vi "Monitoring task.vi"   [LabVIEW 2022 SP3]
uses:
  PLC/PLC.lvlib
types:
  T1 = cluster{bool, "测试模式":enum16{"水样测试", "平行样测试", "集成干预测试", "加标回收"}}
  T2 = typedef "启动参数.ctl" = cluster{"氨氮":bool, "总磷":bool, "总氮":bool, "多参数":bool, "CODmn":bool, "CODCr":bool, "氟化物":bool, "超标留样":bool, "重金属":bool, "挥发酚":bool, "综合生物毒性":bool}
  T3 = cluster{"控制命令":enum16{"启动测量", "标样核查", "零点核查", "跨度核查", "空白测试", "平行样测试", "加标回收", "空白校准", "标样校准", "初始化（清洗）", "停止测试", "仪器重启", "校时", "模式设置", "测量间隔设置"}, "自动运行启动参数":T2}
  T4 = typedef "参数.ctl" = cluster{"测试模式":enum16{"水样测试", "平行样测试", "集成干预测试", "加标回收"}, "参数启用":T2}
  T5 = enum16{"空闲", "润洗", "采样", "沉淀", "配水", "反冲洗", "储水", "结束"}
  T6 = typedef "控制命令与参数.ctl" = cluster{"控制命令":enum16{"启动测量", "标样核查", "零点核查", "跨度核查", "空白测试", "平行样测试", "加标回收", "空白校准", "标样校准", "初始化（清洗）", "停止测试", "仪器重启", "校时", "模式设置", "测量间隔设置"}, "测量参数":string}
  T7 = enum16{"启动测量", "标样核查", "零点核查", "跨度核查", "空白测试", "平行样测试", "加标回收", "空白校准", "标样校准", "初始化（清洗）", "停止测试", "仪器重启", "校时", "模式设置", "测量间隔设置"}
  T8 = typedef "斯坦道原位多参数.lvlib/水样测试启动自定义输入参数.ctl" = cluster{"测量模式":string, "数据类型":string}
  T9 = typedef "多参数模块版本.ctl" = enum16{"原位多参数", "集成式多参"}
  T10 = cluster{"系统时间":timestamp, "工作状态":u16, "测量模式":u16, "告警代码":enum16{"无告警", "缺试剂告警", "缺水样告警", "缺蒸馏水告警", "缺标液告警", "仪表漏液告警", "标定异常告警", "超量程告警", "加热异常", "低试剂预警", "超上限告警", "超下限告警", "仪表内部其他异常", "滴定异常告警", "电极异常告警", "量程切换告警", "参数设置告警", "PH电极电位异常", "电导率电极异常", "浊度光度异常", "溶解氧电极异常", "溶解氧光强异常", "温度异常告警", "PH异常告警", "溶解氧异常告警", "电导率异常告警", "浊度异常告警", "叶绿素异常告警", "藻密度异常告警", "蓝绿藻异常告警", "ORP异常告警", "氨氮异常告警", "清洁刷异常告警", "SD卡异常告警", "蓝牙异常告警", "Wifi异常告警", "流程异常告警"}, "故障代码":enum16{"无故障", "电机故障", "温度故障", "通讯故障", "滴定故障"}, "日志代码":u16, "软件版本":string}
  T11 = cluster{"命令":string, "测量模式":enum16{"水样测量", "标样核查", "零点核查", "跨度核查", "空白测试", "加标回收", "平行样", "校零", "校标"}, "CODMn量程切换":enum32{"H", "L", "AUTO"}}
  T12 = enum16{"水样测量", "标样核查", "零点核查", "跨度核查", "空白测试", "加标回收", "平行样", "校零", "校标"}
  T13 = typedef "模块配置类型.ctl" = enum16{"单模块", "总磷总氮二合一模块", "氨氮总磷二合一模块"}
  T14 = typedef "CODMn模块版本.ctl" = enum16{"PLC版", "单片机版", "通用流路版本"}
  T15 = typedef "CODcr模块版本.ctl" = enum16{"斯坦道V3", "点创"}
  T16 = typedef "氨氮总磷总氮模块版本.ctl" = enum16{"V2", "V3"}
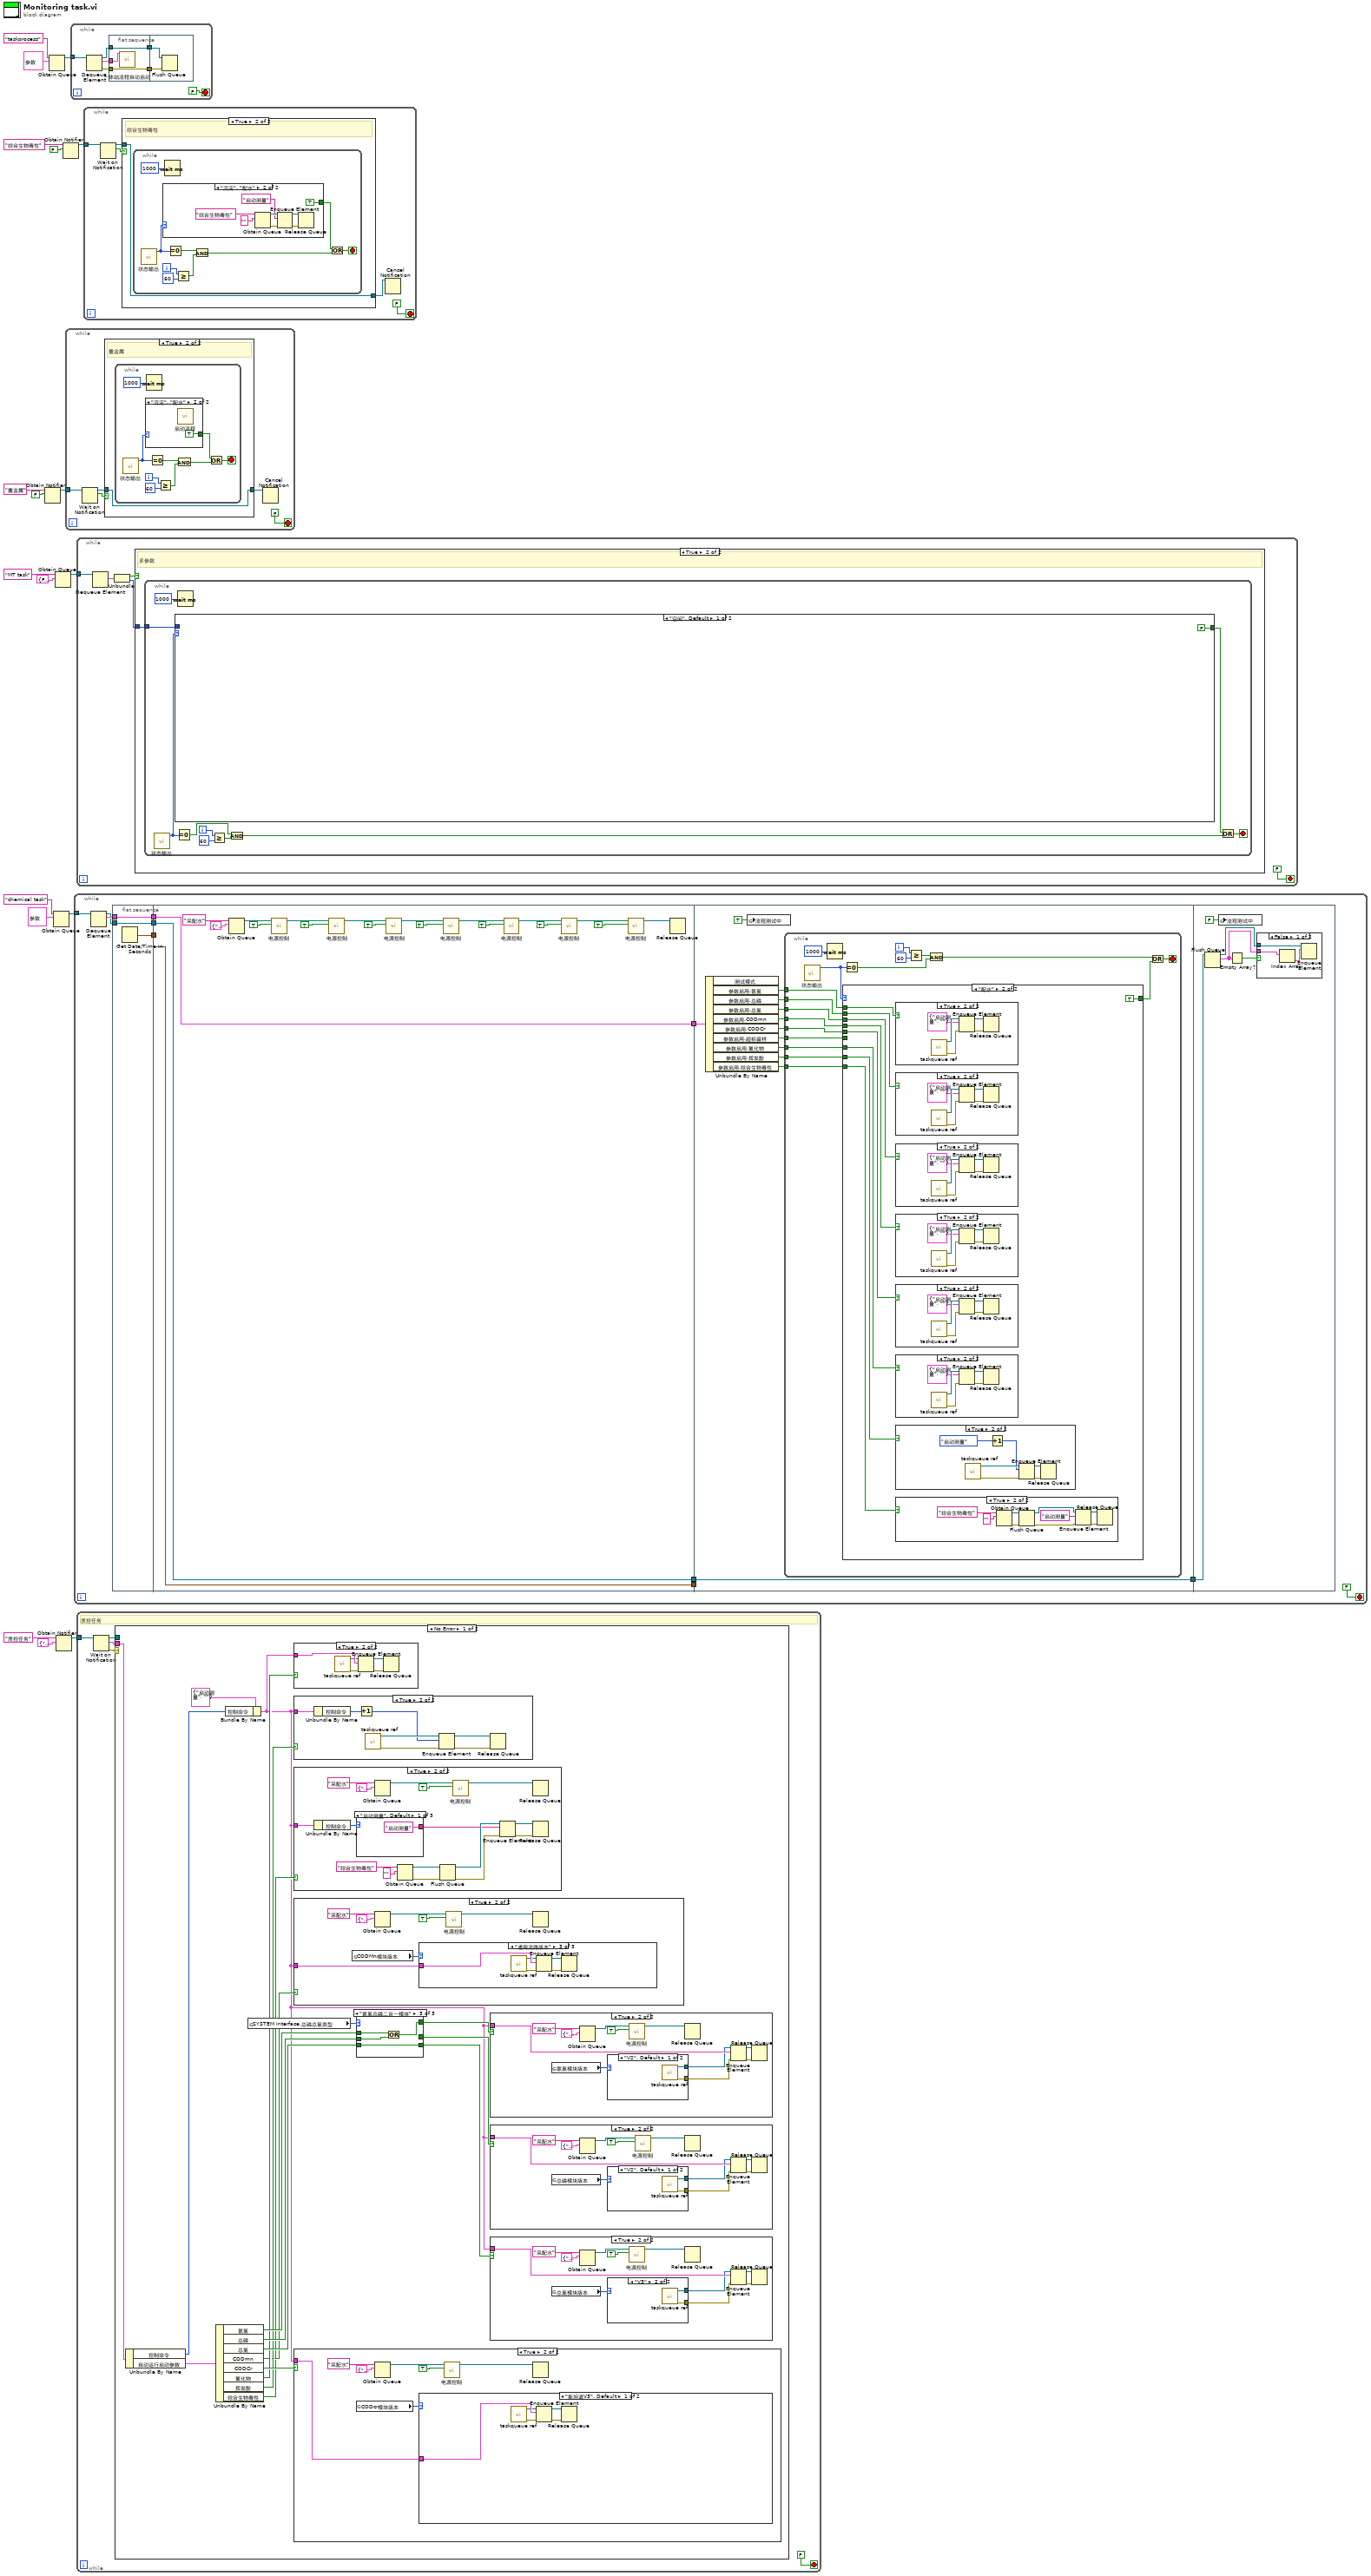
[diagram p0: block diagram]
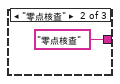
[diagram p7: hidden frame]
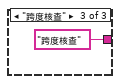
[diagram p8: hidden frame]
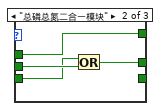
[diagram p12: hidden frame]
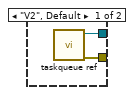
[diagram p14: hidden frame]
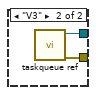
[diagram p16: hidden frame]
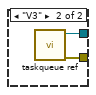
[diagram p18: hidden frame]
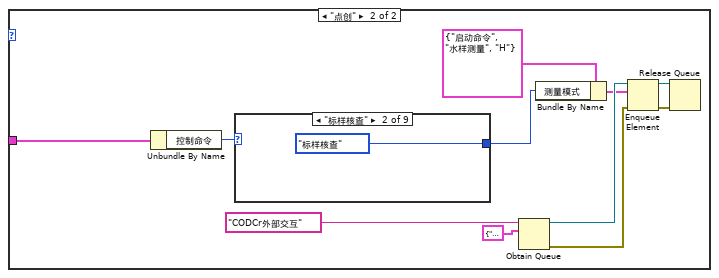
[diagram p20: hidden frame]
diagram:
  n1 = Obtain Notifier(name (unnamed)="重金属" ("名称（未命名）"), notification data type=FALSE) -> (notifier out=w5:refnum<notifier>)  [unwired: 2 in, 2 out]
  n2 = Obtain Queue(name (unnamed)="taskprocess" ("名称（未命名）"), element data type=T4 {"测试模式"=enum."水样测试", "参数启用"={"氨氮"=FALSE, "总磷"=FALSE, "总氮"=FALSE, "多参数"=FALSE, "CODmn"=FALSE, "CODCr"=FALSE, "氟化物"=FALSE, "超标留样"=FALSE, "重金属"=FALSE, "挥发酚"=FALSE, "综合生物毒性"=FALSE}} ("参数")) -> (queue out=w13:refnum<queue>)  [unwired: 3 in, 2 out]
  n3 = Obtain Queue(name (unnamed)="chemical task" ("名称（未命名）"), element data type=T4 {"测试模式"=enum."水样测试", "参数启用"={"氨氮"=FALSE, "总磷"=FALSE, "总氮"=FALSE, "多参数"=FALSE, "CODmn"=FALSE, "CODCr"=FALSE, "氟化物"=FALSE, "超标留样"=FALSE, "重金属"=FALSE, "挥发酚"=FALSE, "综合生物毒性"=FALSE}} ("参数")) -> (queue out=w17:refnum<queue>)  [unwired: 3 in, 2 out]
  n4 = Obtain Queue(name (unnamed)="MT task" ("名称（未命名）"), element data type=T1 {FALSE, "测试模式"=enum."水样测试"}) -> (queue out=w15:refnum<queue>)  [unwired: 3 in, 2 out]
  n5 = Obtain Notifier(name (unnamed)="质控任务" ("名称（未命名）"), notification data type=T3 {"控制命令"=enum."启动测量", "自动运行启动参数"={"氨氮"=FALSE, "总磷"=FALSE, "总氮"=FALSE, "多参数"=FALSE, "CODmn"=FALSE, "CODCr"=FALSE, "氟化物"=FALSE, "超标留样"=FALSE, "重金属"=FALSE, "挥发酚"=FALSE, "综合生物毒性"=FALSE}}) -> (notifier out=w11:refnum<notifier>)  [unwired: 2 in, 2 out]
  n6 = Obtain Notifier(name (unnamed)="综合生物毒性" ("名称（未命名）"), notification data type=FALSE) -> (notifier out=w3:refnum<notifier>)  [unwired: 2 in, 2 out]
  n7 = while {
    tunnel: w5 -> [w23]
    stop <- FALSE stop-if-true
    n8 = Wait on Notification(notifier=w23) -> (notifier out=w20:refnum<notifier>, notification=w22:bool)  [unwired: 3 in, 2 out]
    n9 = case shown="True" w22 {
      tunnel: w20 -> [w24 w25]
      tunnel: [w24 w25] -> w19
      frame False {
      }
      frame True {
        # "重金属"
        n10 = while {
          i -> [w33]
          stop <- w28 stop-if-true
          n11 = call "状态输出.vi"() -> ("采配水流程"=w26:T5)  [unwired: 11 in]
          n12 = case shown="\"沉淀\", \"配水\"" w26 {
            tunnel: [_ TRUE] -> w27
            frame "空闲", Default {
            }
            frame "沉淀", "配水" {
              n13 = call "启动流程.vi"() -> ()  [unwired: 12 in]
            }
          }
          n14 = Wait (ms)(milliseconds to wait=u32 1000 ("等待时间（毫秒）")) -> ()  [unwired: 1 out]
          n15 = Equal To 0?(x=w26) -> (x = 0?=w30:bool)
          n16 = Greater Or Equal?(x=w33, y=60) -> (x >= y?=w31:bool)
          n17 = And(x=w30, y=w31) -> (x .and. y?=w29:bool)
          n18 = Or(x=w27, y=w29) -> (x .or. y?=w28:bool)
        }
      }
    }
    n19 = Cancel Notification(0:w19) -> ()  [unwired: 1 in, 3 out]
  }
  n20 = while {
    tunnel: w13 -> [w42]
    stop <- FALSE stop-if-true
    n21 = Dequeue Element(queue=w42) -> (queue out=w40:refnum<queue>, element=w36:T4, error out=w39:errorcluster)  [unwired: 2 in, 1 out]
    n22 = flat-sequence {
      tunnel: w39 -> [w44]
      tunnel: w40 -> [w45]
      tunnel: [w45] -> w38
      tunnel: [w44] -> w37
      tunnel: w36 -> [w43]
      tunnel: w38 -> [w47]
      tunnel: w37 -> [w46]
      frame #0 {
        n23 = call "一体站流程自动启动.vi"("参数"=w43) -> ()  [unwired: 11 in]
      }
      frame #1 {
        n24 = Flush Queue(queue=w47, error in (no error)=w46) -> ()  [unwired: 3 out]
      }
    }
  }
  n25 = while {
    tunnel: w17 -> [w58]
    stop <- FALSE stop-if-true
    n26 = Dequeue Element(queue=w58) -> (queue out=w53:refnum<queue>, element=w57:T4)  [unwired: 2 in, 2 out]
    n27 = flat-sequence {
      tunnel: w53 -> [w60]
      tunnel: w57 -> [w61]
      tunnel: [w61] -> w51
      tunnel: [w60] -> w50
      tunnel: [w59] -> w49
      tunnel: [w81] -> w55
      tunnel: [w66] -> w54
      tunnel: w51 -> [w81]
      tunnel: w50 -> [w66]
      tunnel: w49 -> [w65]
      tunnel: [w65] -> w48
      tunnel: w55 -> [w93]
      tunnel: w54 -> [w92]
      tunnel: [w92] -> w52
      tunnel: w48 -> [_]
      tunnel: w52 -> [w170]
      frame #0 {
        n28 = Get Date/Time In Seconds() -> (seconds since 1Jan1904=w59:timestamp)
      }
      frame #1 {
        n29 = Obtain Queue(name (unnamed)="采配水" ("名称（未命名）"), element data type=cluster{"命令":string, "数据":variant} {"命令"="", "数据"=variant}) -> (queue out=w78:refnum<queue>)  [unwired: 3 in, 2 out]
        n30 = call-poly "电源控制.vi"("通电/断电"=TRUE, "队列"=w78) -> ("队列输出"=w72:refnum<queue>)  [unwired: 9 in]
        n31 = call-poly "电源控制.vi"("通电/断电"=TRUE, "队列"=w72) -> ("队列输出"=w73:refnum<queue>)  [unwired: 9 in]
        n32 = call-poly "电源控制.vi"("通电/断电"=TRUE, "队列"=w73) -> ("队列输出"=w74:refnum<queue>)  [unwired: 9 in]
        n33 = call-poly "电源控制.vi"("通电/断电"=TRUE, "队列"=w74) -> ("队列输出"=w75:refnum<queue>)  [unwired: 9 in]
        n34 = call-poly "电源控制.vi"("通电/断电"=TRUE, "队列"=w75) -> ("队列输出"=w76:refnum<queue>)  [unwired: 9 in]
        n35 = call-poly "电源控制.vi"("通电/断电"=TRUE, "队列"=w76) -> ("队列输出"=w63:refnum<queue>)  [unwired: 9 in]
        n36 = call-poly "电源控制.vi"("通电/断电"=TRUE, "队列"=w63) -> ("队列输出"=w62:refnum<queue>)  [unwired: 9 in]
        n37 = Release Queue(queue=w62) -> ()  [unwired: 2 in, 3 out]
      }
      frame #2 {
        n38 = Unbundle By Name(w93) -> ("参数启用.氨氮"=w90:bool, "参数启用.总磷"=w89:bool, "参数启用.总氮"=w88:bool, "参数启用.CODmn"=w87:bool, "参数启用.CODCr"=w86:bool, "参数启用.超标留样"=w85:bool, "参数启用.氟化物"=w84:bool, "参数启用.挥发酚"=w83:bool, "参数启用.综合生物毒性"=w82:bool)  [unwired: 1 out]
        n39 = global write "系统设置全局变量.vi" "流程测试中"(TRUE ("流程测试中")) -> ()
        n40 = while {
          tunnel: w90 -> [w107]
          tunnel: w89 -> [w106]
          tunnel: w88 -> [w100]
          tunnel: w87 -> [w99]
          tunnel: w86 -> [w98]
          tunnel: w85 -> [w97]
          tunnel: w84 -> [w96]
          tunnel: w83 -> [w95]
          tunnel: w82 -> [w94]
          i -> [w111]
          stop <- w103 stop-if-true
          n41 = call "状态输出.vi"() -> ("采配水流程"=w105:T5)  [unwired: 11 in]
          n42 = Wait (ms)(milliseconds to wait=u32 1000 ("等待时间（毫秒）")) -> ()  [unwired: 1 out]
          n43 = case shown="\"配水\"" w105 {
            tunnel: w107 -> [_ w120]
            tunnel: w106 -> [_ w119]
            tunnel: [_ TRUE] -> w102
            tunnel: w100 -> [_ w117]
            tunnel: w99 -> [_ w116]
            tunnel: w98 -> [_ w115]
            tunnel: w97 -> [_ _]
            tunnel: w96 -> [_ w112]
            tunnel: w95 -> [_ w113]
            tunnel: w94 -> [_ w114]
            frame "空闲", Default {
            }
            frame "配水" {
              n44 = case shown="True" w120 {
                frame False {
                }
                frame True {
                  n45 = call "taskqueue ref.vi"() -> ("错误输出"=w157:errorcluster, "队列输出"=w158:refnum<queue>)  [unwired: 10 in]
                  n46 = Enqueue Element(queue=w158, element=T6 {"控制命令"=enum."启动测量", "测量参数"=""}, error in (no error)=w157) -> (queue out=w159:refnum<queue>, error out=w160:errorcluster)  [unwired: 1 in, 1 out]
                  n47 = Release Queue(queue=w159, error in (no error)=w160) -> ()  [unwired: 1 in, 3 out]
                }
              }
              n48 = case shown="True" w119 {
                frame False {
                }
                frame True {
                  n49 = call "taskqueue ref.vi"() -> ("错误输出"=w162:errorcluster, "队列输出"=w163:refnum<queue>)  [unwired: 10 in]
                  n50 = Enqueue Element(queue=w163, element=T6 {"控制命令"=enum."启动测量", "测量参数"=""}, error in (no error)=w162) -> (queue out=w165:refnum<queue>, error out=w164:errorcluster)  [unwired: 1 in, 1 out]
                  n51 = Release Queue(queue=w165, error in (no error)=w164) -> ()  [unwired: 1 in, 3 out]
                }
              }
              n52 = case shown="True" w117 {
                frame False {
                }
                frame True {
                  n53 = call "taskqueue ref.vi"() -> ("错误输出"=w152:errorcluster, "队列输出"=w153:refnum<queue>)  [unwired: 10 in]
                  n54 = Enqueue Element(queue=w153, element=T6 {"控制命令"=enum."启动测量", "测量参数"=""}, error in (no error)=w152) -> (queue out=w155:refnum<queue>, error out=w154:errorcluster)  [unwired: 1 in, 1 out]
                  n55 = Release Queue(queue=w155, error in (no error)=w154) -> ()  [unwired: 1 in, 3 out]
                }
              }
              n56 = case shown="True" w116 {
                frame False {
                }
                frame True {
                  n57 = call "taskqueue ref.vi"() -> ("错误输出"=w147:errorcluster, "队列输出"=w148:refnum<queue>)  [unwired: 10 in]
                  n58 = Enqueue Element(queue=w148, element=T6 {"控制命令"=enum."启动测量", "测量参数"=""}, error in (no error)=w147) -> (queue out=w150:refnum<queue>, error out=w149:errorcluster)  [unwired: 1 in, 1 out]
                  n59 = Release Queue(queue=w150, error in (no error)=w149) -> ()  [unwired: 1 in, 3 out]
                }
              }
              n60 = case shown="True" w115 {
                frame False {
                }
                frame True {
                  n61 = call "taskqueue ref.vi"() -> ("错误输出"=w142:errorcluster, "队列输出"=w143:refnum<queue>)  [unwired: 10 in]
                  n62 = Enqueue Element(queue=w143, element=T6 {"控制命令"=enum."启动测量", "测量参数"=""}, error in (no error)=w142) -> (queue out=w144:refnum<queue>, error out=w145:errorcluster)  [unwired: 1 in, 1 out]
                  n63 = Release Queue(queue=w144, error in (no error)=w145) -> ()  [unwired: 1 in, 3 out]
                }
              }
              n64 = case shown="True" w112 {
                frame False {
                }
                frame True {
                  n65 = call "taskqueue ref.vi"() -> ("错误输出"=w122:errorcluster, "队列输出"=w123:refnum<queue>)  [unwired: 10 in]
                  n66 = Enqueue Element(queue=w123, element=T6 {"控制命令"=enum."启动测量", "测量参数"=""}, error in (no error)=w122) -> (queue out=w125:refnum<queue>, error out=w124:errorcluster)  [unwired: 1 in, 1 out]
                  n67 = Release Queue(queue=w125, error in (no error)=w124) -> ()  [unwired: 1 in, 3 out]
                }
              }
              n68 = case shown="True" w113 {
                frame False {
                }
                frame True {
                  n69 = call "taskqueue ref.vi"() -> ("错误输出"=w128:errorcluster, "队列输出"=w129:refnum<queue>)  [unwired: 10 in]
                  n70 = Increment(x=T7."启动测量" ("控制命令")) -> (x+1=w126:T7)
                  n71 = Enqueue Element(queue=w129, element=w126, error in (no error)=w128) -> (queue out=w131:refnum<queue>, error out=w130:errorcluster)  [unwired: 1 in, 1 out]
                  n72 = Release Queue(queue=w131, error in (no error)=w130) -> ()  [unwired: 1 in, 3 out]
                }
              }
              n73 = case shown="True" w114 {
                frame False {
                }
                frame True {
                  n74 = Obtain Queue(name (unnamed)="综合生物毒性" ("名称（未命名）"), element data type="" ("状态")) -> (queue out=w135:refnum<queue>, error out=w136:errorcluster)  [unwired: 3 in, 1 out]
                  n75 = Flush Queue(queue=w135, error in (no error)=w136) -> (queue out=w139:refnum<queue>, error out=w140:errorcluster)  [unwired: 1 out]
                  n76 = Enqueue Element(queue=w139, element="启动测量" ("名称（未命名）"), error in (no error)=w140) -> (queue out=w137:refnum<queue>, error out=w138:errorcluster)  [unwired: 1 in, 1 out]
                  n77 = Release Queue(queue=w137, error in (no error)=w138) -> ()  [unwired: 1 in, 3 out]
                }
              }
            }
          }
          n78 = Equal To 0?(x=w105) -> (x = 0?=w104:bool)
          n79 = Greater Or Equal?(x=w111, y=60) -> (x >= y?=w109:bool)
          n80 = And(x=w109, y=w104) -> (x .and. y?=w108:bool)
          n81 = Or(x=w108, y=w102) -> (x .or. y?=w103:bool)
        }
      }
      frame #3 {
        n82 = Flush Queue(queue=w170) -> (queue out=w169:refnum<queue>, remaining elements=w168:T4[])  [unwired: 1 in, 1 out]
        n83 = global write "系统设置全局变量.vi" "流程测试中"(FALSE ("流程测试中")) -> ()
        n84 = Empty Array?(array=w168) -> (empty?=w167:bool)
        n85 = case shown="False" w167 {
          tunnel: w169 -> [w172 _]
          tunnel: w168 -> [w171 _]
          frame False {
            n86 = Index Array(array=w171) -> (element=w173:T4)  [unwired: 1 in]
            n87 = Enqueue Element(queue=w172, element=w173) -> ()  [unwired: 2 in, 3 out]
          }
          frame True {
          }
        }
      }
    }
  }
  n88 = while {
    tunnel: w15 -> [w178]
    stop <- FALSE stop-if-true
    n89 = Dequeue Element(queue=w178) -> (element=w176:T1)  [unwired: 2 in, 3 out]
    n90 = Unbundle(w176) -> (w175:bool, "测试模式"=w174:enum16{"水样测试", "平行样测试", "集成干预测试", "加标回收"})
    n91 = case shown="True" w175 {
      tunnel: w174 -> [_ w179]
      frame False {
        (unwired) TRUE ("t")
      }
      frame True {
        # "多参数"
        n92 = while {
          tunnel: w179 -> [w189]
          i -> [w180]
          stop <- w184 stop-if-true
          n93 = call "状态输出.vi"() -> ("采配水流程"=w182:T5)  [unwired: 11 in]
          n94 = case shown="\"空闲\", Default" w182 {
            tunnel: w189 -> [_ w192]
            tunnel: [FALSE w191] -> w183
            frame "空闲", Default {
            }
            frame "沉淀", "配水" {
              n95 = case shown="\"水样测试\", Default" w192 {
                tunnel: [TRUE TRUE] -> w191
                frame "水样测试", Default {
                  n96 = flat-sequence {
                    tunnel: [w201] -> w200
                    tunnel: w200 -> [w207]
                    tunnel: [w207] -> w199
                    tunnel: [w206] -> w198
                    tunnel: w199 -> [w222]
                    tunnel: w198 -> [w221]
                    tunnel: [w222] -> w197
                    tunnel: [w221] -> w196
                    tunnel: w197 -> [w224]
                    tunnel: w196 -> [w223]
                    tunnel: [w224] -> w195
                    tunnel: w195 -> [w234]
                    tunnel: [w234] -> w194
                    tunnel: w194 -> [w236]
                    frame #0 {
                      n97 = Obtain Queue(name (unnamed)="采配水" ("名称（未命名）"), element data type=cluster{"命令":string, "数据":variant} {"命令"="", "数据"=variant}) -> (queue out=w203:refnum<queue>)  [unwired: 3 in, 2 out]
                      n98 = call-poly "电源控制.vi"("通电/断电"=TRUE, "队列"=w203) -> ("队列输出"=w201:refnum<queue>)  [unwired: 9 in]
                    }
                    frame #1 {
                      n99 = global read "系统设置全局变量.vi" "运行模式"() -> (w209:enum16{"维护模式", "常规模式", "应急模式", "质控模式"})
                      n100 = case shown="\"维护模式\"" w209 {
                        tunnel: ["M" ("数据标记表") "N" ("数据标记表")] -> w208
                        frame "维护模式" {
                        }
                        frame "常规模式", Default {
                        }
                      }
                      n101 = global read "系统设置全局变量.vi" "多参数模块版本"() -> (w206:T9)
                      n102 = case shown="\"集成式多参\"" w206 {
                        tunnel: w208 -> [w212 w217]
                        frame "原位多参数", Default {
                          n103 = Bundle By Name(cluster=T8 {"测量模式"="水样测试", "数据类型"="N"} ("元素"), "数据类型"=w212) -> (w213:T8)
                          n104 = call "taskqueue ref.vi"() -> ("队列输出"=w211:refnum<queue>)  [unwired: 10 in, 1 out]
                          n105 = Enqueue Element(queue=w211, element=w213) -> (queue out=w210:refnum<queue>)  [unwired: 2 in, 2 out]
                          n106 = Release Queue(queue=w210) -> ()  [unwired: 2 in, 3 out]
                        }
                        frame "集成式多参" {
                          n107 = call "taskqueue ref.vi"() -> ("队列输出"=w216:refnum<queue>)  [unwired: 10 in, 1 out]
                          n108 = Enqueue Element(queue=w216, element=w217) -> (queue out=w215:refnum<queue>)  [unwired: 2 in, 2 out]
                          n109 = Release Queue(queue=w215) -> ()  [unwired: 2 in, 3 out]
                        }
                      }
                    }
                    frame #2 {
                      n110 = Wait (ms)(milliseconds to wait=u32 5000) -> ()  [unwired: 1 out]
                    }
                    frame #3 {
                      n111 = while {
                        tunnel: w223 -> [w227]
                        stop <- w226 stop-if-true
                        n112 = case shown="\"集成式多参\"" w227 {
                          tunnel: [w228 w231] -> w226
                          frame "原位多参数", Default {
                            n113 = global read "多参数全局变量.vi" "状态告警区"() -> (w230:T10)
                            n114 = Unbundle By Name(w230) -> ("工作状态"=w229:u16)
                            n115 = Equal To 0?(x=w229) -> (x = 0?=w228:bool)
                          }
                          frame "集成式多参" {
                            n116 = global read "多参数全局变量.vi" "多参数运行状态"() -> (w232:u16)
                            n117 = Equal To 0?(x=w232) -> (x = 0?=w231:bool)
                          }
                        }
                        n118 = Wait (ms)(milliseconds to wait=u32 1000) -> ()  [unwired: 1 out]
                      }
                    }
                    frame #4 {
                      n119 = Wait (ms)(milliseconds to wait=u32 5000) -> ()  [unwired: 1 out]
                    }
                    frame #5 {
                      n120 = call-poly "电源控制.vi"("通电/断电"=FALSE, "队列"=w236) -> ("队列输出"=w235:refnum<queue>)  [unwired: 9 in]
                      n121 = Release Queue(queue=w235) -> ()  [unwired: 2 in, 3 out]
                    }
                  }
                }
                frame "集成干预测试" {
                  n122 = global read "系统设置全局变量.vi" "运行模式"() -> (w241:enum16{"维护模式", "常规模式", "应急模式", "质控模式"})
                  n123 = case shown="\"常规模式\", Default" w241 {
                    tunnel: ["M" ("数据标记表") "N" ("数据标记表")] -> w240
                    frame "维护模式" {
                    }
                    frame "常规模式", Default {
                    }
                  }
                  n124 = global read "系统设置全局变量.vi" "多参数模块版本"() -> (w239:T9)
                  n125 = case shown="\"集成式多参\"" w239 {
                    tunnel: w240 -> [w245 w249]
                    frame "原位多参数", Default {
                      n126 = Bundle By Name(cluster=T8 {"测量模式"="水样测试", "数据类型"="N"} ("元素"), "数据类型"=w245) -> (w242:T8)
                      n127 = call "taskqueue ref.vi"() -> ("队列输出"=w243:refnum<queue>)  [unwired: 10 in, 1 out]
                      n128 = Enqueue Element(queue=w243, element=w242) -> (queue out=w244:refnum<queue>)  [unwired: 2 in, 2 out]
                      n129 = Release Queue(queue=w244) -> ()  [unwired: 2 in, 3 out]
                    }
                    frame "集成式多参" {
                      n130 = call "JCGYtaskqueue ref.vi"() -> ("队列输出"=w247:refnum<queue>)  [unwired: 10 in, 1 out]
                      n131 = Enqueue Element(queue=w247, element=w249) -> (queue out=w248:refnum<queue>)  [unwired: 2 in, 2 out]
                      n132 = Release Queue(queue=w248) -> ()  [unwired: 2 in, 3 out]
                    }
                  }
                }
              }
            }
          }
          n133 = Equal To 0?(x=w182) -> (x = 0?=w186:bool)
          n134 = Wait (ms)(milliseconds to wait=u32 1000 ("等待时间（毫秒）")) -> ()  [unwired: 1 out]
          n135 = Greater Or Equal?(x=w180, y=60) -> (x >= y?=w187:bool)
          n136 = And(x=w186, y=w187) -> (x .and. y?=w185:bool)
          n137 = Or(x=w183, y=w185) -> (x .or. y?=w184:bool)
        }
      }
    }
  }
  n138 = while {
    tunnel: w11 -> [w256]
    stop <- FALSE stop-if-true
    # "质控任务"
    n139 = Wait on Notification(notifier=w256) -> (notifier out=w252:refnum<notifier>, notification=w254:T3, error out=w253:errorcluster)  [unwired: 3 in, 1 out]
    n140 = case shown="No Error" w253 {
      tunnel: w254 -> [w264 _]
      tunnel: w252 -> [_ _]
      frame No Error {
        n141 = Unbundle By Name(w264) -> ("控制命令"=w260:T7, "自动运行启动参数"=w263:T2)
        n142 = Unbundle By Name(w263) -> ("氨氮"=w267:bool, "总磷"=w269:bool, "总氮"=w271:bool, "CODmn"=w259:bool, "CODCr"=w273:bool, "氟化物"=w265:bool, "挥发酚"=w262:bool, "综合生物毒性"=w258:bool)
        n143 = Bundle By Name(cluster=T6 {"控制命令"=enum."启动测量", "测量参数"=""} ("输入参数"), "控制命令"=w260) -> (w257:T6)
        n144 = global read "系统设置全局变量.vi" "SYSTEM Interface.总磷总氮类型"() -> (w272:T13)
        n145 = case shown="True" w265 {
          tunnel: w257 -> [_ w302]
          frame False {
          }
          frame True {
            n146 = call "taskqueue ref.vi"() -> ("错误输出"=w300:errorcluster, "队列输出"=w301:refnum<queue>)  [unwired: 10 in]
            n147 = Enqueue Element(queue=w301, element=w302, error in (no error)=w300) -> (queue out=w304:refnum<queue>, error out=w303:errorcluster)  [unwired: 1 in, 1 out]
            n148 = Release Queue(queue=w304, error in (no error)=w303) -> ()  [unwired: 1 in, 3 out]
          }
        }
        n149 = case shown="True" w262 {
          tunnel: w257 -> [_ w295]
          frame False {
          }
          frame True {
            n150 = Unbundle By Name(w295) -> ("控制命令"=w293:T7)
            n151 = Increment(x=w293) -> (x+1=w294:T7)
            n152 = call "taskqueue ref.vi"() -> ("错误输出"=w296:errorcluster, "队列输出"=w297:refnum<queue>)  [unwired: 10 in]
            n153 = Enqueue Element(queue=w297, element=w294, error in (no error)=w296) -> (queue out=w299:refnum<queue>, error out=w298:errorcluster)  [unwired: 1 in, 1 out]
            n154 = Release Queue(queue=w299, error in (no error)=w298) -> ()  [unwired: 1 in, 3 out]
          }
        }
        n155 = case shown="True" w258 {
          tunnel: w257 -> [_ w289]
          frame False {
          }
          frame True {
            n156 = Unbundle By Name(w289) -> ("控制命令"=w279:T7)
            n157 = case shown="\"启动测量\", Default" w279 {
              tunnel: ["启动测量" ("名称（未命名）") "零点核查" ("名称（未命名）") "跨度核查" ("名称（未命名）")] -> w280
              frame "启动测量", Default {
              }
              frame "零点核查" {
              }
              frame "跨度核查" {
              }
            }
            n158 = Obtain Queue(name (unnamed)="采配水" ("名称（未命名）"), element data type=cluster{"命令":string, "数据":variant} {"命令"="", "数据"=variant}) -> (queue out=w276:refnum<queue>)  [unwired: 3 in, 2 out]
            n159 = Obtain Queue(name (unnamed)="综合生物毒性" ("名称（未命名）"), element data type="" ("状态")) -> (queue out=w283:refnum<queue>, error out=w284:errorcluster)  [unwired: 3 in, 1 out]
            n160 = Flush Queue(queue=w283, error in (no error)=w284) -> (queue out=w287:refnum<queue>, error out=w288:errorcluster)  [unwired: 1 out]
            n161 = call-poly "电源控制.vi"("通电/断电"=TRUE, "队列"=w276) -> ("队列输出"=w275:refnum<queue>)  [unwired: 9 in]
            n162 = Enqueue Element(queue=w287, element=w280, error in (no error)=w288) -> (queue out=w285:refnum<queue>, error out=w286:errorcluster)  [unwired: 1 in, 1 out]
            n163 = Release Queue(queue=w275) -> ()  [unwired: 2 in, 3 out]
            n164 = Release Queue(queue=w285, error in (no error)=w286) -> ()  [unwired: 1 in, 3 out]
          }
        }
        n165 = case shown="True" w259 {
          tunnel: w257 -> [_ w399]
          frame False {
          }
          frame True {
            n166 = global read "系统设置全局变量.vi" "CODMn模块版本"() -> (w393:T14)
            n167 = Obtain Queue(name (unnamed)="采配水" ("名称（未命名）"), element data type=cluster{"命令":string, "数据":variant} {"命令"="", "数据"=variant}) -> (queue out=w396:refnum<queue>)  [unwired: 3 in, 2 out]
            n168 = case shown="\"通用流路版本\"" w393 {
              tunnel: w399 -> [w403 w410 w415]
              frame "PLC版", Default {
                n169 = Unbundle By Name(w403) -> ("控制命令"=w400:T7)
                n170 = call "taskqueue ref.vi"() -> ("错误输出"=w401:errorcluster, "队列输出"=w402:refnum<queue>)  [unwired: 10 in]
                n171 = Enqueue Element(queue=w402, element=w400, error in (no error)=w401) -> (queue out=w405:refnum<queue>, error out=w404:errorcluster)  [unwired: 1 in, 1 out]
                n172 = Release Queue(queue=w405, error in (no error)=w404) -> ()  [unwired: 1 in, 3 out]
              }
              frame "单片机版" {
                n173 = Unbundle By Name(w410) -> ("控制命令"=w406:T7)
                n174 = Increment(x=w406) -> (x+1=w407:T7)
                n175 = call "taskqueue ref.vi"() -> ("错误输出"=w408:errorcluster, "队列输出"=w409:refnum<queue>)  [unwired: 10 in]
                n176 = Enqueue Element(queue=w409, element=w407, error in (no error)=w408) -> (queue out=w412:refnum<queue>, error out=w411:errorcluster)  [unwired: 1 in, 1 out]
                n177 = Release Queue(queue=w412, error in (no error)=w411) -> ()  [unwired: 1 in, 3 out]
              }
              frame "通用流路版本" {
                n178 = call "taskqueue ref.vi"() -> ("错误输出"=w413:errorcluster, "队列输出"=w414:refnum<queue>)  [unwired: 10 in]
                n179 = Enqueue Element(queue=w414, element=w415, error in (no error)=w413) -> (queue out=w417:refnum<queue>, error out=w416:errorcluster)  [unwired: 1 in, 1 out]
                n180 = Release Queue(queue=w417, error in (no error)=w416) -> ()  [unwired: 1 in, 3 out]
              }
            }
            n181 = call-poly "电源控制.vi"("通电/断电"=TRUE, "队列"=w396) -> ("队列输出"=w397:refnum<queue>)  [unwired: 9 in]
            n182 = Release Queue(queue=w397) -> ()  [unwired: 2 in, 3 out]
          }
        }
        n183 = case shown="True" w273 {
          tunnel: w257 -> [_ w367]
          frame False {
          }
          frame True {
            n184 = global read "系统设置全局变量.vi" "CODcr模块版本"() -> (w361:T15)
            n185 = Obtain Queue(name (unnamed)="采配水" ("名称（未命名）"), element data type=cluster{"命令":string, "数据":variant} {"命令"="", "数据"=variant}) -> (queue out=w364:refnum<queue>)  [unwired: 3 in, 2 out]
            n186 = case shown="\"斯坦道V3\", Default" w361 {
              tunnel: w367 -> [w370 w374]
              frame "斯坦道V3", Default {
                n187 = call "taskqueue ref.vi"() -> ("错误输出"=w368:errorcluster, "队列输出"=w369:refnum<queue>)  [unwired: 10 in]
                n188 = Enqueue Element(queue=w369, element=w370, error in (no error)=w368) -> (queue out=w371:refnum<queue>, error out=w372:errorcluster)  [unwired: 1 in, 1 out]
                n189 = Release Queue(queue=w371, error in (no error)=w372) -> ()  [unwired: 1 in, 3 out]
              }
              frame "点创" {
                n190 = Unbundle By Name(w374) -> ("控制命令"=w373:T7)
                n191 = case shown="\"标样核查\"" w373 {
                  tunnel: [T12."水样测量" ("测量模式") T12."标样核查" ("测量模式") T12."零点核查" ("测量模式") T12."跨度核查" ("测量模式") T12."空白测试" ("测量模式") T12."平行样" ("测量模式") T12."加标回收" ("测量模式") T12."校零" ("测量模式") T12."校标" ("测量模式")] -> w383
                  frame "启动测量", Default {
                  }
                  frame "标样核查" {
                  }
                  frame "零点核查" {
                  }
                  frame "跨度核查" {
                  }
                  frame "空白测试" {
                  }
                  frame "平行样测试" {
                  }
                  frame "加标回收" {
                  }
                  frame "空白校准" {
                  }
                  frame "标样校准" {
                  }
                }
                n192 = Obtain Queue(name (unnamed)="CODCr外部交互" ("名称（未命名）"), element data type=T11 {"命令"="启动命令", "测量模式"=enum."水样测量", "CODMn量程切换"=enum."AUTO"} ("元素")) -> (queue out=w381:refnum<queue>, error out=w382:errorcluster)  [unwired: 3 in, 1 out]
                n193 = Bundle By Name(cluster=T11 {"命令"="启动命令", "测量模式"=enum."水样测量", "CODMn量程切换"=enum."H"} ("元素"), "测量模式"=w383) -> (w380:T11)
                n194 = Enqueue Element(queue=w381, element=w380, error in (no error)=w382) -> (queue out=w377:refnum<queue>, error out=w378:errorcluster)  [unwired: 1 in, 1 out]
                n195 = Release Queue(queue=w377, error in (no error)=w378) -> ()  [unwired: 1 in, 3 out]
              }
            }
            n196 = call-poly "电源控制.vi"("通电/断电"=TRUE, "队列"=w364) -> ("队列输出"=w365:refnum<queue>)  [unwired: 9 in]
            n197 = Release Queue(queue=w365) -> ()  [unwired: 2 in, 3 out]
          }
        }
        n198 = case shown="\"氨氮总磷二合一模块\"" w272 {
          tunnel: [w307 _ w315] -> w270
          tunnel: w271 -> [w307 w309 w315]
          tunnel: w269 -> [w306 w310 w314]
          tunnel: [w306 w311 _] -> w268
          tunnel: w267 -> [w305 w308 w313]
          tunnel: [w305 w308 w312] -> w266
          frame "单模块", Default {
          }
          frame "总磷总氮二合一模块" {
            n199 = Or(x=w309, y=w310) -> (x .or. y?=w311:bool)
          }
          frame "氨氮总磷二合一模块" {
            n200 = Or(x=w313, y=w314) -> (x .or. y?=w312:bool)
          }
        }
        n201 = case shown="True" w266 {
          tunnel: w257 -> [_ w339]
          frame False {
          }
          frame True {
            n202 = global read "系统设置全局变量.vi" "氨氮模块版本"() -> (w331:T16)
            n203 = Obtain Queue(name (unnamed)="采配水" ("名称（未命名）"), element data type=cluster{"命令":string, "数据":variant} {"命令"="", "数据"=variant}) -> (queue out=w336:refnum<queue>)  [unwired: 3 in, 2 out]
            n204 = case shown="\"V2\", Default" w331 {
              tunnel: [w343 w345] -> w333
              tunnel: [w342 w344] -> w332
              frame "V2", Default {
                n205 = call "taskqueue ref.vi"() -> ("错误输出"=w342:errorcluster, "队列输出"=w343:refnum<queue>)  [unwired: 10 in]
              }
              frame "V3" {
                n206 = call "taskqueue ref.vi"() -> ("错误输出"=w344:errorcluster, "队列输出"=w345:refnum<queue>)  [unwired: 10 in]
              }
            }
            n207 = call-poly "电源控制.vi"("通电/断电"=TRUE, "队列"=w336) -> ("队列输出"=w337:refnum<queue>)  [unwired: 9 in]
            n208 = Release Queue(queue=w337) -> ()  [unwired: 2 in, 3 out]
            n209 = Enqueue Element(queue=w333, element=w339, error in (no error)=w332) -> (queue out=w340:refnum<queue>, error out=w341:errorcluster)  [unwired: 1 in, 1 out]
            n210 = Release Queue(queue=w340, error in (no error)=w341) -> ()  [unwired: 1 in, 3 out]
          }
        }
        n211 = case shown="True" w268 {
          tunnel: w257 -> [_ w354]
          frame False {
          }
          frame True {
            n212 = global read "系统设置全局变量.vi" "总磷模块版本"() -> (w346:T16)
            n213 = Obtain Queue(name (unnamed)="采配水" ("名称（未命名）"), element data type=cluster{"命令":string, "数据":variant} {"命令"="", "数据"=variant}) -> (queue out=w351:refnum<queue>)  [unwired: 3 in, 2 out]
            n214 = case shown="\"V2\", Default" w346 {
              tunnel: [w358 w360] -> w348
              tunnel: [w357 w359] -> w347
              frame "V2", Default {
                n215 = call "taskqueue ref.vi"() -> ("错误输出"=w357:errorcluster, "队列输出"=w358:refnum<queue>)  [unwired: 10 in]
              }
              frame "V3" {
                n216 = call "taskqueue ref.vi"() -> ("错误输出"=w359:errorcluster, "队列输出"=w360:refnum<queue>)  [unwired: 10 in]
              }
            }
            n217 = call-poly "电源控制.vi"("通电/断电"=TRUE, "队列"=w351) -> ("队列输出"=w352:refnum<queue>)  [unwired: 9 in]
            n218 = Release Queue(queue=w352) -> ()  [unwired: 2 in, 3 out]
            n219 = Enqueue Element(queue=w348, element=w354, error in (no error)=w347) -> (queue out=w356:refnum<queue>, error out=w355:errorcluster)  [unwired: 1 in, 1 out]
            n220 = Release Queue(queue=w356, error in (no error)=w355) -> ()  [unwired: 1 in, 3 out]
          }
        }
        n221 = case shown="True" w270 {
          tunnel: w257 -> [_ w324]
          frame False {
          }
          frame True {
            n222 = global read "系统设置全局变量.vi" "总氮模块版本"() -> (w316:T16)
            n223 = Obtain Queue(name (unnamed)="采配水" ("名称（未命名）"), element data type=cluster{"命令":string, "数据":variant} {"命令"="", "数据"=variant}) -> (queue out=w321:refnum<queue>)  [unwired: 3 in, 2 out]
            n224 = case shown="\"V3\"" w316 {
              tunnel: [w328 w330] -> w318
              tunnel: [w327 w329] -> w317
              frame "V2", Default {
                n225 = call "taskqueue ref.vi"() -> ("错误输出"=w327:errorcluster, "队列输出"=w328:refnum<queue>)  [unwired: 10 in]
              }
              frame "V3" {
                n226 = call "taskqueue ref.vi"() -> ("错误输出"=w329:errorcluster, "队列输出"=w330:refnum<queue>)  [unwired: 10 in]
              }
            }
            n227 = call-poly "电源控制.vi"("通电/断电"=TRUE, "队列"=w321) -> ("队列输出"=w322:refnum<queue>)  [unwired: 9 in]
            n228 = Release Queue(queue=w322) -> ()  [unwired: 2 in, 3 out]
            n229 = Enqueue Element(queue=w318, element=w324, error in (no error)=w317) -> (queue out=w326:refnum<queue>, error out=w325:errorcluster)  [unwired: 1 in, 1 out]
            n230 = Release Queue(queue=w326, error in (no error)=w325) -> ()  [unwired: 1 in, 3 out]
          }
        }
      }
      frame Error {
      }
    }
  }
  n231 = while {
    tunnel: w3 -> [w422]
    stop <- FALSE stop-if-true
    n232 = Wait on Notification(notifier=w422) -> (notifier out=w419:refnum<notifier>, notification=w421:bool)  [unwired: 3 in, 2 out]
    n233 = case shown="True" w421 {
      tunnel: w419 -> [w423 w424]
      tunnel: [w423 w424] -> w418
      frame False {
      }
      frame True {
        # "综合生物毒性"
        n234 = while {
          i -> [w432]
          stop <- w427 stop-if-true
          n235 = call "状态输出.vi"() -> ("采配水流程"=w425:T5)  [unwired: 11 in]
          n236 = case shown="\"沉淀\", \"配水\"" w425 {
            tunnel: [_ TRUE] -> w426
            frame "空闲", Default {
            }
            frame "沉淀", "配水" {
              n237 = Obtain Queue(name (unnamed)="综合生物毒性" ("名称（未命名）"), element data type="" ("状态")) -> (queue out=w437:refnum<queue>, error out=w438:errorcluster)  [unwired: 3 in, 1 out]
              n238 = Enqueue Element(queue=w437, element="启动测量" ("名称（未命名）"), error in (no error)=w438) -> (queue out=w439:refnum<queue>, error out=w440:errorcluster)  [unwired: 1 in, 1 out]
              n239 = Release Queue(queue=w439, error in (no error)=w440) -> ()  [unwired: 1 in, 3 out]
            }
          }
          n240 = Wait (ms)(milliseconds to wait=u32 1000 ("等待时间（毫秒）")) -> ()  [unwired: 1 out]
          n241 = Equal To 0?(x=w425) -> (x = 0?=w429:bool)
          n242 = Greater Or Equal?(x=w432, y=60) -> (x >= y?=w430:bool)
          n243 = And(x=w429, y=w430) -> (x .and. y?=w428:bool)
          n244 = Or(x=w426, y=w428) -> (x .or. y?=w427:bool)
        }
      }
    }
    n245 = Cancel Notification(0:w418) -> ()  [unwired: 1 in, 3 out]
  }
